vi "Map Function.vi"(6 "Ysup":dbl=5.0, 8 "Yinf":dbl=5.0, 9 "Xsup":dbl, 10 "Xinf":dbl, 11 "X":dbl) -> (2 "Value":dbl)   [LabVIEW 2012]
doc: "Este VI mapeia a variável X com intervalo [Xinf, Xsup] para o respectivo valor no intervalo [Yinf, Ysup]."
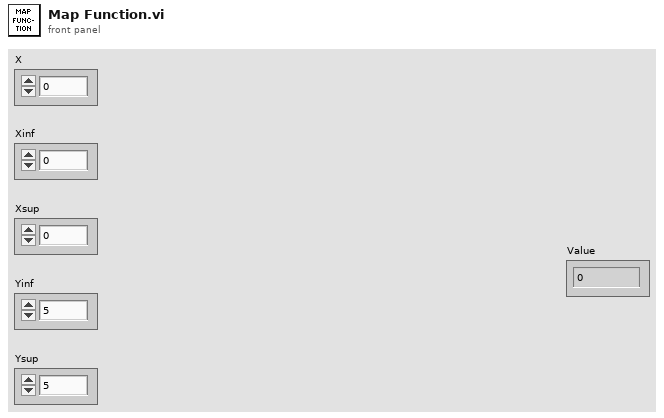
[diagram p1: front panel]
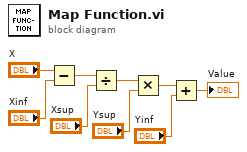
[diagram p0: block diagram]
diagram:
  n1 = Subtract(x="X", y="Xinf") -> (x-y=w8:dbl)
  n2 = Divide(x=w8, y="Xsup") -> (x/y=w6:dbl)
  n3 = Multiply(x=w6, y="Ysup") -> (x*y=w3:dbl)
  n4 = Add(x=w3, y="Yinf") -> (x+y=→"Value":dbl)
